vi "VIP_Pre-Install Custom Action.vi"(10 "Variant":variant) -> (0 "error out":errorcluster)   [LabVIEW 2020]
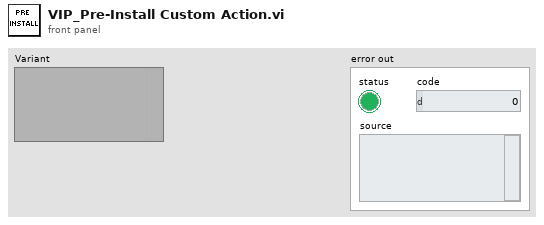
[diagram p1: front panel]
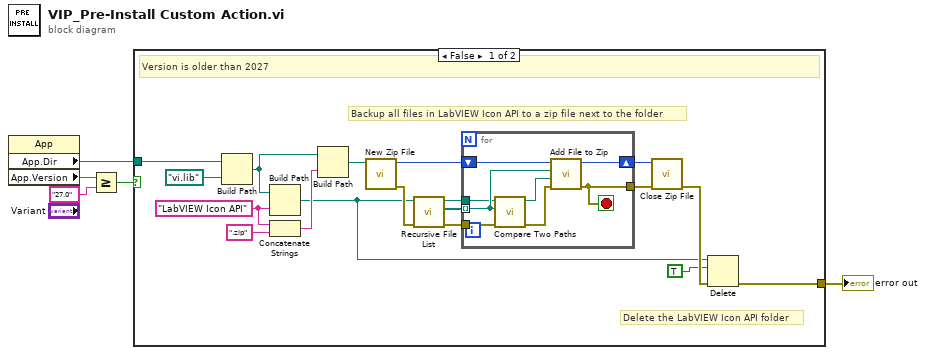
[diagram p0: block diagram]
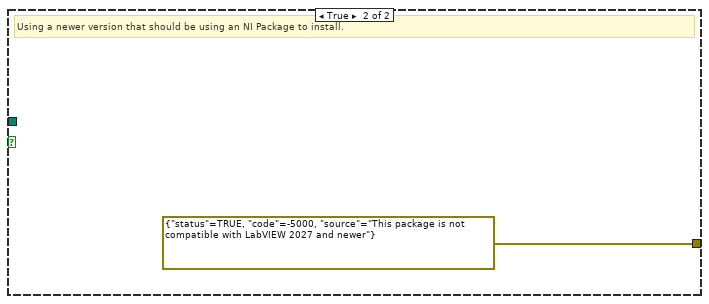
[diagram p2: hidden frame]
diagram:
  n1 = property class="App"() -> ("App.Dir"=w1:path, "App.Version"=w4:string)  [unwired: 2 in, 2 out]
  n2 = Greater Or Equal?(x=w4, y="27.0") -> (x >= y?=w2:bool)
  n3 = case shown="False" w2 {
    tunnel: [w19 errorcluster {"status"=TRUE, "code"=-5000, "source"="This package is not compatible with LabVIEW 2027 and newer"} ("error constant")] -> w5
    tunnel: w1 -> [w6 _]
    frame False {
      w12 = "LabVIEW Icon API"
      # "Delete the LabVIEW Icon API folder"
      # "Backup all files in LabVIEW Icon API to a zip file next to the folder"
      # "Version is older than 2027"
      n4 = Build Path(base path=w6, name or relative path=path "vi.lib" ("symbolic path")) -> (appended path=w10:path)
      n5 = Build Path(base path=w10, name or relative path=w12) -> (appended path=w7:path)
      n6 = Concatenate Strings(w12, ".zip" ("string")) -> (w9:string)
      n7 = Build Path(base path=w10, name or relative path=w9) -> (appended path=w8:path)
      n8 = call <vilib>:"New Zip File.vi"("target"=w8) -> ("error out"=w20:errorcluster, "zip file out"=w16:i64)  [unwired: 4 in, 1 out]
      n9 = call <vilib>:"Recursive File List.vi"("error in (no error)"=w20, "Folder Path"=w7) -> ("error out"=w21:errorcluster, "All Files in Dir"=w18:path[], "dup Folder Path"=w14:path)  [unwired: 5 in, 2 out]
      n10 = for {
        tunnel: w18 -> [w26] mode=indexing
        tunnel: w21 -> [w30]
        tunnel: [w31] -> w22
        shift-right: [w27] -> w17
        shift-left: w16 -> [w28]
        tunnel: w14 -> [w25]
        stop <- w31 stop-if-true
        n11 = call <vilib>:"Compare Two Paths.vi"("error in (no error)"=w30, "Path 2"=w26, "Path 1"=w25) -> ("error out"=w29:errorcluster, "Relative Path from 1 to 2"=w24:path)  [unwired: 5 in, 2 out]
        n12 = call <vilib>:"Add File to Zip.vi"("error in (no error)"=w29, "destination path in zip"=w24, "source file path"=w26, "zip file in"=w28) -> ("error out"=w31:errorcluster, "zip file out"=w27:i64)  [unwired: 6 out]
      }
      n13 = call <vilib>:"Close Zip File.vi"("error in (no error)"=w22, "zip file in"=w17) -> ("error out"=w23:errorcluster)  [unwired: 5 in]
      n14 = Delete(path (use dialog)=w7, entire hierarchy (F)=TRUE, error in=w23) -> (error out=w19:errorcluster)  [unwired: 2 in, 2 out]
    }
    frame True {
      # "Using a newer version that should be using an NI Package to install."
    }
  }
  "error out" <- w5
